vi "Initialize Instrument.vi"(8 "error in (no error)":errorcluster, 10 "Reset":bool, 11 "SA-ESA in":refnum<class "SA-ESA.lvclass">) -> (0 "error out":errorcluster, 3 "SA-ESA out":refnum<class "SA-ESA.lvclass">)   [LabVIEW 2020, in "SA-ESA.lvclass"]
doc: "Initilization of the ESA spectrum analyzer"
uses:
  SA-ESA.lvclass
  C:/Sandbox/RF Bench/Source Code/WiSpry Test Framework/Instruments/Instrument.lvclass
  C:/Sandbox/RF Bench/Source Code/WiSpry Test Framework/Instruments/Spectrum Analyzer/Spectrum Analyzer.lvclass
  Instrument.lvclass/Instrument.ctl
  Spectrum Analyzer.lvclass/Spectrum Analyzer.ctl
  <vilib>/Utility/config.llb/Read Key (Double).vi
  Instrument.lvclass
  Spectrum Analyzer.lvclass
  <vilib>/Utility/config.llb/NI_LVConfig.lvlib
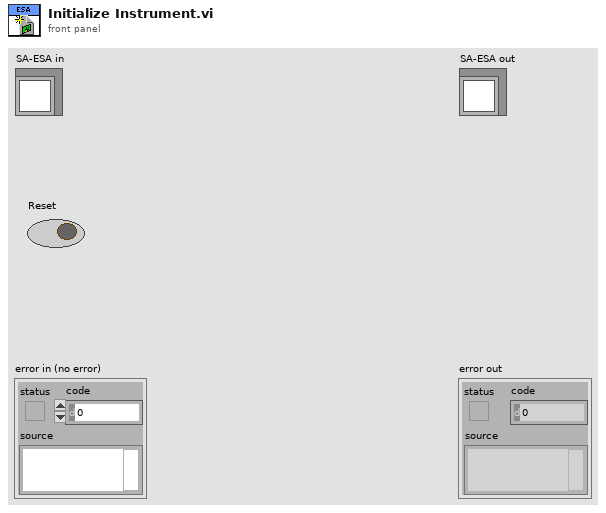
[diagram p1: front panel]
types:
  T1 = typedef "NI_LVConfig.lvlib/Config Data RefNum.ctl" = refnum<k1>
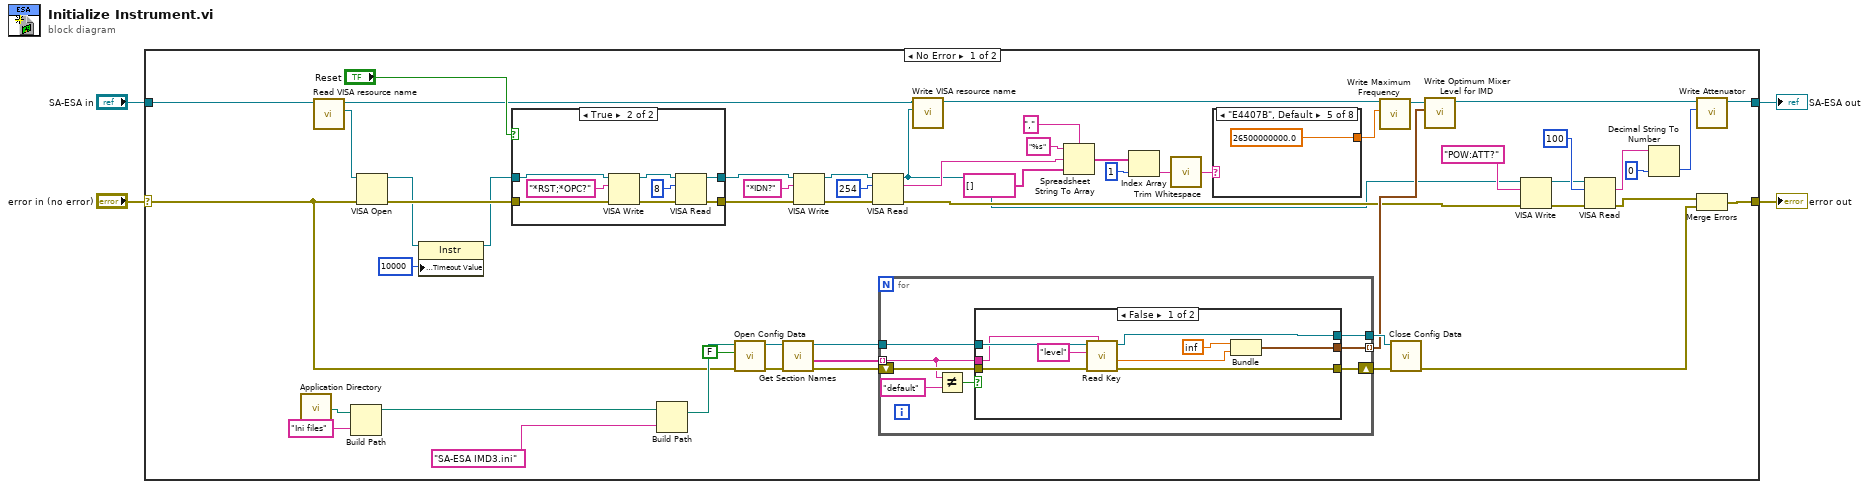
[diagram p0: block diagram]
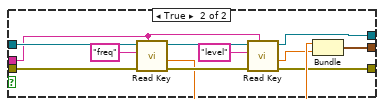
[diagram p2: hidden frame]
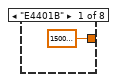
[diagram p3: hidden frame]
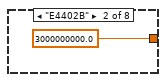
[diagram p4: hidden frame]
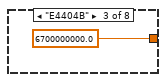
[diagram p5: hidden frame]
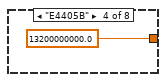
[diagram p6: hidden frame]
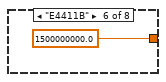
[diagram p7: hidden frame]
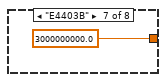
[diagram p8: hidden frame]
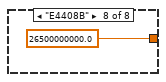
[diagram p9: hidden frame]
diagram:
  n1 = case shown="No Error" "error in (no error)" {
    selector: "error in (no error)" -> [w27 w106]
    tunnel: "SA-ESA in" -> [w58 w107]
    tunnel: [w26 w106] -> w2
    tunnel: [w6 w107] -> w1
    frame No Error {
      n2 = call <vilib>:"Application Directory.vi"() -> ("Application Directory"=w39:path)
      n3 = call "Read VISA resource name.vi"("Instrument in"=w58) -> ("VISA resource name"=w57:refnum<visa-resource-name>, "Instrument out"=w21:refnum<class "SA-ESA.lvclass">)  [unwired: 9 in]
      n4 = Build Path(base path=w39, name or relative path="Ini files") -> (appended path=w38:path)
      n5 = VISA Open(error in (no error)=w27, VISA resource name=w57) -> (VISA resource name=w18:refnum<visa-resource-name>, error out=w55:errorcluster)  [unwired: 3 in]
      n6 = property class="Instr"(reference=w18, "General Settings:Timeout Value"=u32 10000) -> (reference out=w17:refnum<visa-resource-name>)  [unwired: 1 in, 1 out]
      n7 = case shown="True" "Reset" {
        tunnel: w17 -> [w97 w104]
        tunnel: w55 -> [w96 w105]
        tunnel: [w96 w98] -> w54
        tunnel: [w97 w99] -> w53
        frame False {
        }
        frame True {
          n8 = VISA Write(VISA resource name=w104, write buffer="*RST;*OPC?", error in (no error)=w105) -> (VISA resource name out=w101:refnum<visa-resource-name>, error out=w102:errorcluster)  [unwired: 1 out]
          n9 = VISA Read(VISA resource name=w101, byte count=u32 8, error in (no error)=w102) -> (VISA resource name out=w99:refnum<visa-resource-name>, error out=w98:errorcluster)  [unwired: 2 out]
        }
      }
      n10 = Build Path(base path=w38, name or relative path="SA-ESA IMD3.ini") -> (appended path=w29:path)
      n11 = call <vilib>:"Open Config Data.vi"("error in (no error)"=w27, "create file if necessary (T)"=FALSE, "configuration file path"=w29) -> ("error out"=w36:errorcluster, "refnum"=w35:T1)  [unwired: 6 in, 1 out]
      n12 = call <vilib>:"Get Section Names.vi"("error in (no error)"=w36, "refnum"=w35) -> ("error out"=w34:errorcluster, "section names"=w33:string[], "refnum out"=w32:T1)  [unwired: 7 in]
      n13 = VISA Write(VISA resource name=w53, write buffer="*IDN?", error in (no error)=w54) -> (VISA resource name out=w50:refnum<visa-resource-name>, error out=w51:errorcluster)  [unwired: 1 out]
      n14 = VISA Read(VISA resource name=w50, byte count=u32 254, error in (no error)=w51) -> (VISA resource name out=w10:refnum<visa-resource-name>, read buffer=w48:string, error out=w11:errorcluster)  [unwired: 1 out]
      n15 = for {
        tunnel: w33 -> [w62] mode=indexing
        tunnel: w32 -> [w63]
        shift-right: [w60] -> w31
        shift-left: w34 -> [w64]
        tunnel: [w61] -> w22 mode=indexing
        tunnel: [w59] -> w24
        n16 = Not Equal?(x=w62, y="default") -> (x != y?=w65:bool)
        n17 = case shown="False" w65 {
          tunnel: w64 -> [w75 w87]
          tunnel: w63 -> [w74 w86]
          tunnel: w62 -> [w73 w84]
          tunnel: [w67 w78] -> w61
          tunnel: [w69 w77] -> w60
          tunnel: [w68 w76] -> w59
          frame False {
            n18 = call-poly <vilib>:"Read Key.vi"("section"=w73, "error in (no error)"=w75, "key"="level", "refnum"=w74) -> ("error out"=w69:errorcluster, "value"=w70:dbl, "refnum out"=w68:T1)  [unwired: 4 in, 1 out]
            n19 = Bundle(inf, "value"=w70) -> (w67:cluster{dbl, "value":dbl})  [unwired: 1 in]
          }
          frame True {
            n20 = call-poly <vilib>:"Read Key.vi"("section"=w84, "error in (no error)"=w87, "key"="freq", "refnum"=w86) -> ("error out"=w85:errorcluster, "value"=w80:dbl, "refnum out"=w82:T1)  [unwired: 4 in, 1 out]
            n21 = call-poly <vilib>:"Read Key.vi"("section"=w84, "error in (no error)"=w85, "key"="level", "refnum"=w82) -> ("error out"=w77:errorcluster, "value"=w79:dbl, "refnum out"=w76:T1)  [unwired: 4 in, 1 out]
            n22 = Bundle("value"=w80, "value"=w79) -> (w78:cluster{"value":dbl, "value":dbl})  [unwired: 1 in]
          }
        }
      }
      n23 = call "Write VISA resource name.vi"("VISA resource name"=w10, "Instrument in"=w21) -> ("Instrument out"=w20:refnum<class "SA-ESA.lvclass">)  [unwired: 9 in]
      n24 = Spreadsheet String To Array(delimiter (Tab)=",", format string="%s", spreadsheet string=w48, array type (2D Dbl)=string[] []) -> (array=w44:string[])
      n25 = Index Array(array=w44, index=1) -> (element=w42:string)
      n26 = call <vilib>:"Trim Whitespace.vi"("string"=w42) -> ("trimmed string"=w41:string)  [unwired: 1 in]
      n27 = case shown="\"E4407B\", Default" w41 {
        tunnel: [1500000000.0 3000000000.0 6700000000.0 13200000000.0 26500000000.0 1500000000.0 3000000000.0 26500000000.0] -> w40
        frame "E4401B" {
        }
        frame "E4402B" {
        }
        frame "E4404B" {
        }
        frame "E4405B" {
        }
        frame "E4407B", Default {
        }
        frame "E4411B" {
        }
        frame "E4403B" {
        }
        frame "E4408B" {
        }
      }
      n28 = call "Write Maximum Frequency.vi"("Maximum Frequency"=w40, "Spectrum Analyzer in"=w20) -> ("Spectrum Analyzer out"=w23:refnum<class "SA-ESA.lvclass">)  [unwired: 9 in]
      n29 = call <vilib>:"Close Config Data.vi"("error in (no error)"=w31, "refnum"=w24) -> ("error out"=w25:errorcluster)  [unwired: 8 in, 1 out]
      n30 = call "Write Optimum Mixer Level for IMD.vi"("Optimum Mixer Level for IMD"=w22, "Spectrum Analyzer in"=w23) -> ("Spectrum Analyzer out"=w7:refnum<class "SA-ESA.lvclass">)  [unwired: 9 in]
      n31 = VISA Write(VISA resource name=w10, write buffer="POW:ATT?", error in (no error)=w11) -> (VISA resource name out=w13:refnum<visa-resource-name>, error out=w9:errorcluster)  [unwired: 1 out]
      n32 = VISA Read(VISA resource name=w13, byte count=u32 100, error in (no error)=w9) -> (read buffer=w16:string, error out=w8:errorcluster)  [unwired: 2 out]
      n33 = Decimal String To Number(string=w16, default (0L)=u32 0) -> (number=w5:u32)  [unwired: 1 in, 1 out]
      n34 = call "Write Attenuator.vi"("Attenuator"=w5, "Spectrum Analyzer in"=w7) -> ("Spectrum Analyzer out"=w6:refnum<class "SA-ESA.lvclass">)  [unwired: 9 in]
      n35 = Merge Errors(w8, w25) -> (w26:errorcluster)
    }
    frame Error {
    }
  }
  "error out" <- w2
  "SA-ESA out" <- w1
